vi "Log.vi"   [LabVIEW 2019, in "xy_utilities.lvlib"]
doc: "Square <b>XY-data</b>'s y array.\n\nWire data to the data input to determine the polymorphic instance to use or manually select the instance."
uses:
  xy_utilities.lvlib
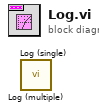
[diagram p0: block diagram]
diagram:
  n1 = call "Log (multiple).vi"() -> ()  [unwired: 10 in, 2 out]
  n2 = call "Log (single).vi"() -> ()  [unwired: 10 in, 2 out]
